vi "Read current pos notifier.vi"(8 "error in (no error)":errorcluster, 11 "MotionSystem Configuration in":refnum<class "MotionSystem Configuration.lvclass">) -> (0 "error out":errorcluster, 2 "current pos notifier":refnum<notifier>, 3 "MotionSystem Configuration out":refnum<class "MotionSystem Configuration.lvclass">)   [LabVIEW 2016, in "MotionSystem.lvlib" / "MotionSystem Configuration.lvclass"]
uses:
  <userlib>/Common Components/Hardware/Abstract System/MotionSystem/MotionSystem Config/MotionSystem Configuration.lvclass
  G:/tasks/labview/Fermi Utility Framework/Functions/RPS-3DOF/Controls/Array of Current Pos.ctl
  <userlib>/Common Components/Hardware/Abstract System/MotionSystem/MotionSystem Config/MotionSystem Configuration.lvclass/MotionSystem Configuration.ctl
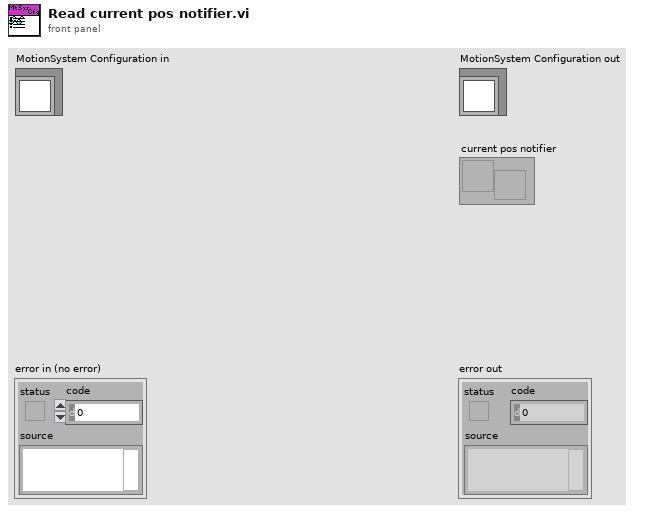
[diagram p1: front panel]
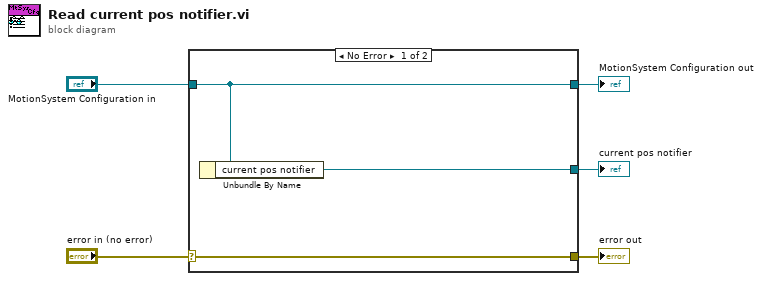
[diagram p0: block diagram]
diagram:
  n1 = case shown="No Error" "error in (no error)" {
    selector: "error in (no error)" -> [w8 w9]
    tunnel: [w8 w9] -> w4
    tunnel: [w7 w10] -> w2
    tunnel: "MotionSystem Configuration in" -> [w7 w10]
    tunnel: [w6 _] -> w1
    frame No Error {
      n2 = Unbundle By Name(w7) -> ("current pos notifier"=w6:refnum<notifier>)
    }
    frame Error {
    }
  }
  "error out" <- w4
  "MotionSystem Configuration out" <- w2
  "current pos notifier" <- w1
